vi "rs232.vi"() -> ()   [LabVIEW 2014]
uses:
  <vilib>/Instr/_visa.llb/VISA Configure Serial Port (Instr).vi
panel:
  in  "string to write":string="*IDN?"
  in  "stop":bool
  in  "read":bool=TRUE
  in  "write":bool=TRUE
  out "read string":string
  out "actual bytes read":u32
  in  "XON Character":u8=17 format="%.0x"
  in  "XOFF Character":u8=19 format="%.0x"
  in  "flow control":u16(ring) items=["None"=0, "XON/XOFF"=1, "RTS/CTS"=2, "DTR/DSR"=4]
  in  "End write with termination character?":bool=TRUE
  in  "termination char\n(0xA = '\\n' = LF)":u8=10 format="%.0x"
  in  "End read on termination character?":bool=TRUE
  in  "timeout (ms)":u32=10000
  in  "stop bits":u16(ring)=10 items=["1.0"=10, "1.5"=15, "2.0"=20]
  in  "parity":u16(ring) items=["None", "Odd", "Even", "Mark", "Space"]
  in  "data bits":u16=8 min=5 max=8 step=1
  in  "VISA resource name":refnum<visa-resource-name>="COM1"
  in  "baud rate":u32=9600
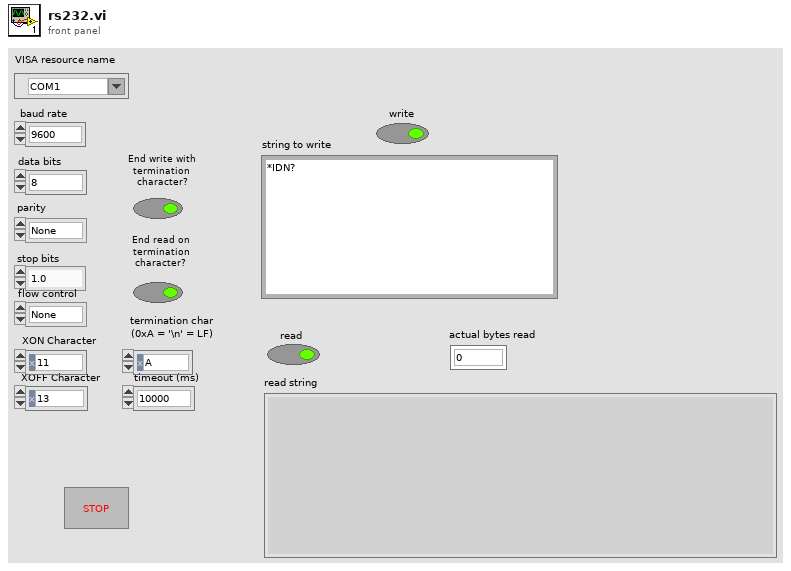
[diagram p1: front panel]
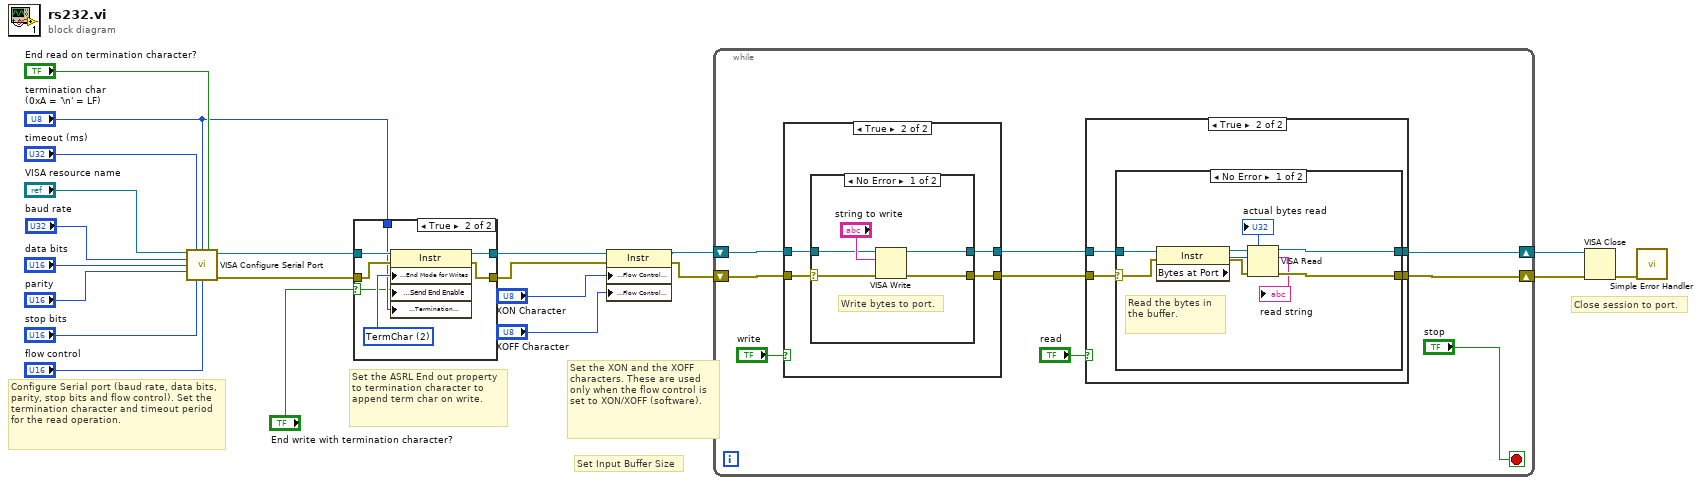
[diagram p0: block diagram]
diagram:
  # "Close session to port."
  # "Set the XON and the XOFF characters. These are used only when the flow control is set to XON/XOFF (software)."
  # "Configure Serial port (baud rate, data bits, parity, stop bits and flow control). Set the termination character and timeout period for the read operation."
  # "Set Input Buffer Size"
  # "Set the ASRL End out property to termination character to append term char on write."
  n1 = call-poly "VISA Configure Serial Port"("VISA resource name"="VISA resource name", "timeout (10sec)"="timeout (ms)", "termination char\n(0xA = '\\n' = LF)"="termination char\n(0xA = '\\n' = LF)", "Enable Termination\nChar (T)"="End read on termination character?", "baud rate (9600)"="baud rate", "data bits (8)"="data bits", "parity (0:none)"="parity", "stop bits (10: 1 bit)"="stop bits", "flow control (0:none)"="flow control") -> ("VISA resource name out"=w8:refnum<visa-resource-name>, "error out"=w9:errorcluster)  [unwired: 1 in, 4 out]
  n2 = case shown="True" "End write with termination character?" {
    selector: "End write with termination character?" -> [_ w24]
    tunnel: w8 -> [w22 w30]
    tunnel: w9 -> [w23 w29]
    tunnel: [w22 w28] -> w7
    tunnel: [w23 w27] -> w6
    tunnel: "termination char\n(0xA = '\\n' = LF)" -> [_ w25]
    frame False {
    }
    frame True {
      w26 = u16 2 items=["None", "LastBit", "TermChar", "Break"] ("Serial Settings:Serial End Mode for Writes")
      n3 = property class="Instr"(reference=w30, error in=w29, "Serial Settings:End Mode for Writes"=w26, "Message Based Settings:Send End Enable"=w24, "Message Based Settings:Termination Character"=w25) -> (reference out=w28:refnum<visa-resource-name>, error out=w27:errorcluster)
    }
  }
  n4 = property class="Instr"(reference=w7, error in=w6, "Serial Settings:Flow Control XON Character"="XON Character", "Serial Settings:Flow Control XOFF Character"="XOFF Character") -> (reference out=w2:refnum<visa-resource-name>, error out=w1:errorcluster)
  n5 = while {
    shift-right: [w35] -> w4
    shift-left: w2 -> [w33]
    shift-right: [w34] -> w3
    shift-left: w1 -> [w32]
    stop <- "stop" stop-if-true
    n6 = case shown="True" "write" {
      tunnel: [w41 w45] -> w38
      tunnel: [w40 w44] -> w37
      tunnel: w33 -> [w41 w43]
      tunnel: w32 -> [w40 w42]
      frame False {
      }
      frame True {
        n7 = case shown="No Error" w42 {
          selector: w42 -> [w46 w52]
          tunnel: [w50 w51] -> w45
          tunnel: [w49 w52] -> w44
          tunnel: w43 -> [w47 w51]
          frame No Error {
            # "Write bytes to port."
            n8 = VISA Write(VISA resource name=w47, write buffer="string to write", error in (no error)=w46) -> (VISA resource name out=w50:refnum<visa-resource-name>, error out=w49:errorcluster)  [unwired: 1 out]
          }
          frame Error {
          }
        }
      }
    }
    n9 = case shown="True" "read" {
      tunnel: w37 -> [w53 w56]
      tunnel: w38 -> [w54 w55]
      tunnel: [w53 w58] -> w34
      tunnel: [w54 w57] -> w35
      frame False {
      }
      frame True {
        n10 = case "Read bytes from port." shown="No Error" w56 {
          selector: w56 -> [w61 w68]
          tunnel: [w66 w68] -> w58
          tunnel: [w67 w69] -> w57
          tunnel: w55 -> [w62 w69]
          frame No Error {
            # "Read the bytes in the buffer."
            n11 = property class="Instr"(reference=w62, error in=w61) -> (reference out=w60:refnum<visa-resource-name>, error out=w59:errorcluster, "Bytes at Port"=w63:u32)
            n12 = VISA Read(VISA resource name=w60, byte count=w63, error in (no error)=w59) -> (VISA resource name out=w67:refnum<visa-resource-name>, read buffer=→"read string":string, return count=→"actual bytes read":u32, error out=w66:errorcluster)
          }
          frame Error {
            # "Error occurred \nreading Bytes at \nSerial Port"
          }
        }
      }
    }
  }
  n13 = VISA Close(VISA resource name=w4, error in (no error)=w3) -> (error out=w5:errorcluster)
  n14 = call <vilib>:"Simple Error Handler.vi"("error in (no error)"=w5) -> ()  [unwired: 1 in, 8 out]
